vi "File path- counter.vi"(9 "Station No":string, 10 "Model Name":string) -> (2 "File Path":path)   [LabVIEW 2015]
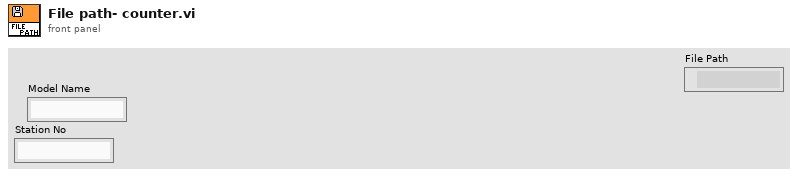
[diagram p1: front panel]
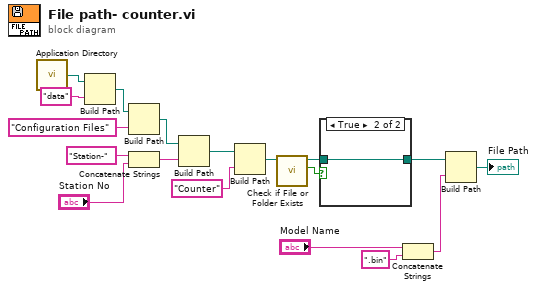
[diagram p0: block diagram]
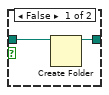
[diagram p2: hidden frame]
diagram:
  n1 = call <vilib>:"Application Directory.vi"() -> ("Application Directory"=w18:path)
  n2 = Build Path(base path=w18, name or relative path="data") -> (appended path=w15:path)
  n3 = Build Path(base path=w15, name or relative path="Configuration Files") -> (appended path=w13:path)
  n4 = Concatenate Strings("Station-" ("string"), "Station No") -> (w9:string)
  n5 = Build Path(base path=w13, name or relative path=w9) -> (appended path=w12:path)
  n6 = Build Path(base path=w12, name or relative path="Counter" ("Folder Name")) -> (appended path=w8:path)
  n7 = call <vilib>:"Check if File or Folder Exists.vi"("path"=w8) -> ("file or folder exists?"=w6:bool, "dup path"=w7:path)  [unwired: 8 in, 1 out]
  n8 = case shown="True" w6 {
    tunnel: w7 -> [w20 w21]
    tunnel: [w19 w21] -> w5
    frame False {
      n9 = Create Folder(path (use dialog)=w20) -> (created path=w19:path)  [unwired: 2 in, 2 out]
    }
    frame True {
    }
  }
  n10 = Concatenate Strings("Model Name", ".bin") -> (w2:string)
  n11 = Build Path(base path=w5, name or relative path=w2) -> (appended path=→"File Path":path)
